vi "Autonomous Independent.vi"() -> ()   [LabVIEW 2014]
doc: "This VI is called when autonomous begins, and will automatically be terminated when autonomous ends. You can carry out timed or sensor driven robot movement independently without needing to return to the caller."
uses:
  <vilib>/Rock Robotics/WPI/RobotDrive/WPI_RobotDriveGetSetRefNum.vi
  <vilib>/Utility/file.llb/Read From Spreadsheet File (DBL).vi
  <vilib>/Rock Robotics/WPI/RobotDrive/WPI_RobotDriveMecanumDrive_Cartesian.vi
  Robot Global Data.vi
panel:
  out "?":dbl[][](array[numeric])
  out "Distance 3":dbl
  out "Distance 2":dbl
  out "Gyro Angle":dbl
  out "Gyro Angle 2":dbl
  out "Distance":bool
  out "Stop":bool
  out "Rotate":bool
  out "Shoot":bool
  out "Pick-up":bool
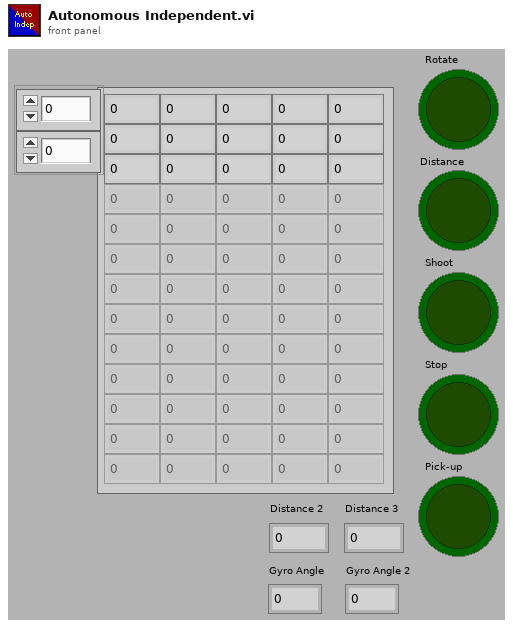
[diagram p1: front panel]
types:
  T1 = typedef "WPI_EncoderDevRef.ctl" = cluster{"DevStatus":errorcluster, "EncoderIndex":T2, "CounterIndex":T3, "DistancePerCount":dbl, "Decoding Type":T4}
  T2 = typedef "FPGA_EncoderIdx.ctl" = enum8{"Enc 0", "Enc 1", "Enc 2", "Enc 3", "Enc 4", "Enc 5", "Enc 6", "Enc 7", "Invalid"}
  T3 = typedef "FPGA_CounterCtrSystemIndex.ctl" = enum8{"Ctr 0", "Ctr 1", "Ctr 2", "Ctr 3", "Ctr 4", "Ctr 5", "Ctr 6", "Ctr 7", "Invalid"}
  T4 = typedef "WPI_EncoderType.ctl" = enum16{"1x", "2x", "4x"}
  T5 = typedef "WPI_RobotDriveDevRef.ctl" = cluster{"DevStatus":errorcluster, "Motors[]":T6[], "Square Inputs":bool, "Max Output":dbl}
  T6 = typedef "WPI_MotorControlDeviceRef.ctl" = cluster{"DeviceStatus":errorcluster, "Type":T7, "PWM":cluster{"Controller":T8, "PWM Channel":T9, "DeadBand":T10}, "CAN":cluster{"Device Number":u8, "Control Mode":T11, "Semaphore":T12, "Max Vout":dbl, "TalonSRX Control Mode":T13}, "Invert":bool, "TransformRef":T14, "InvTransformRef":T14}
  T7 = typedef "WPI_MotorControlType.ctl" = enum16{"PWM", "CAN", "CANTalonSRX"}
  T8 = typedef "FPGA_TypedefDigitalModule.ctl" = enum16{"Controller 1"}
  T9 = typedef "FPGA_DIOPWMChannel.ctl" = enum8{"PWM 0", "PWM 1", "PWM 2", "PWM 3", "PWM 4", "PWM 5", "PWM 6", "PWM 7", "PWM 8", "PWM 9", "PWM MXP 0", "PWM MXP 1", "PWM MXP 2", "PWM MXP 3", "PWM MXP 4", "PWM MXP 5", "PWM MXP 6", "PWM MXP 7", "PWM MXP 8", "PWM MXP 9", "Invalid"}
  T10 = typedef "WPI_PWMDeadband.ctl" = cluster{"Name":string, "maxPositivePwm":i32, "minPositivePwm":i32, "centerPwm":i32, "maxNegativePwm":i32, "minNegativePwm":i32, "angularRange":u16}
  T11 = typedef "WPI_CANJaguar_ControlMode.ctl" = enum8{"Percent VBus", "Current", "Speed", "Position", "Voltage"}
  T12 = typedef "Semaphore RefNum" = refnum<k1>
  T13 = typedef "WPI_CANTalonSRX_APIControlMode.ctl" = enum8{"Percent VBus", "Speed", "Position", "Slave", "Unchanged / Invalid"}
  T14 = typedef "WPI_PWMTransform_ConPane.ctl" = refnum<vi>
  T15 = typedef "WPI_GyroDevRef.ctl" = cluster{"DevStatus":errorcluster, "Analog Module":T16, "Analog Channel":T17, "Offset":dbl, "Gain (VoltsPerDegree/Second)":dbl}
  T16 = typedef "FPGA_TypedefAnalogModule.ctl" = enum16{"Controller 1"}
  T17 = typedef "FPGA_AIChannel.ctl" = enum8{"AI 0", "AI 1", "AI 2", "AI 3", "AI MXP 0", "AI MXP 1", "AI MXP 2", "AI MXP 3", "Invalid"}
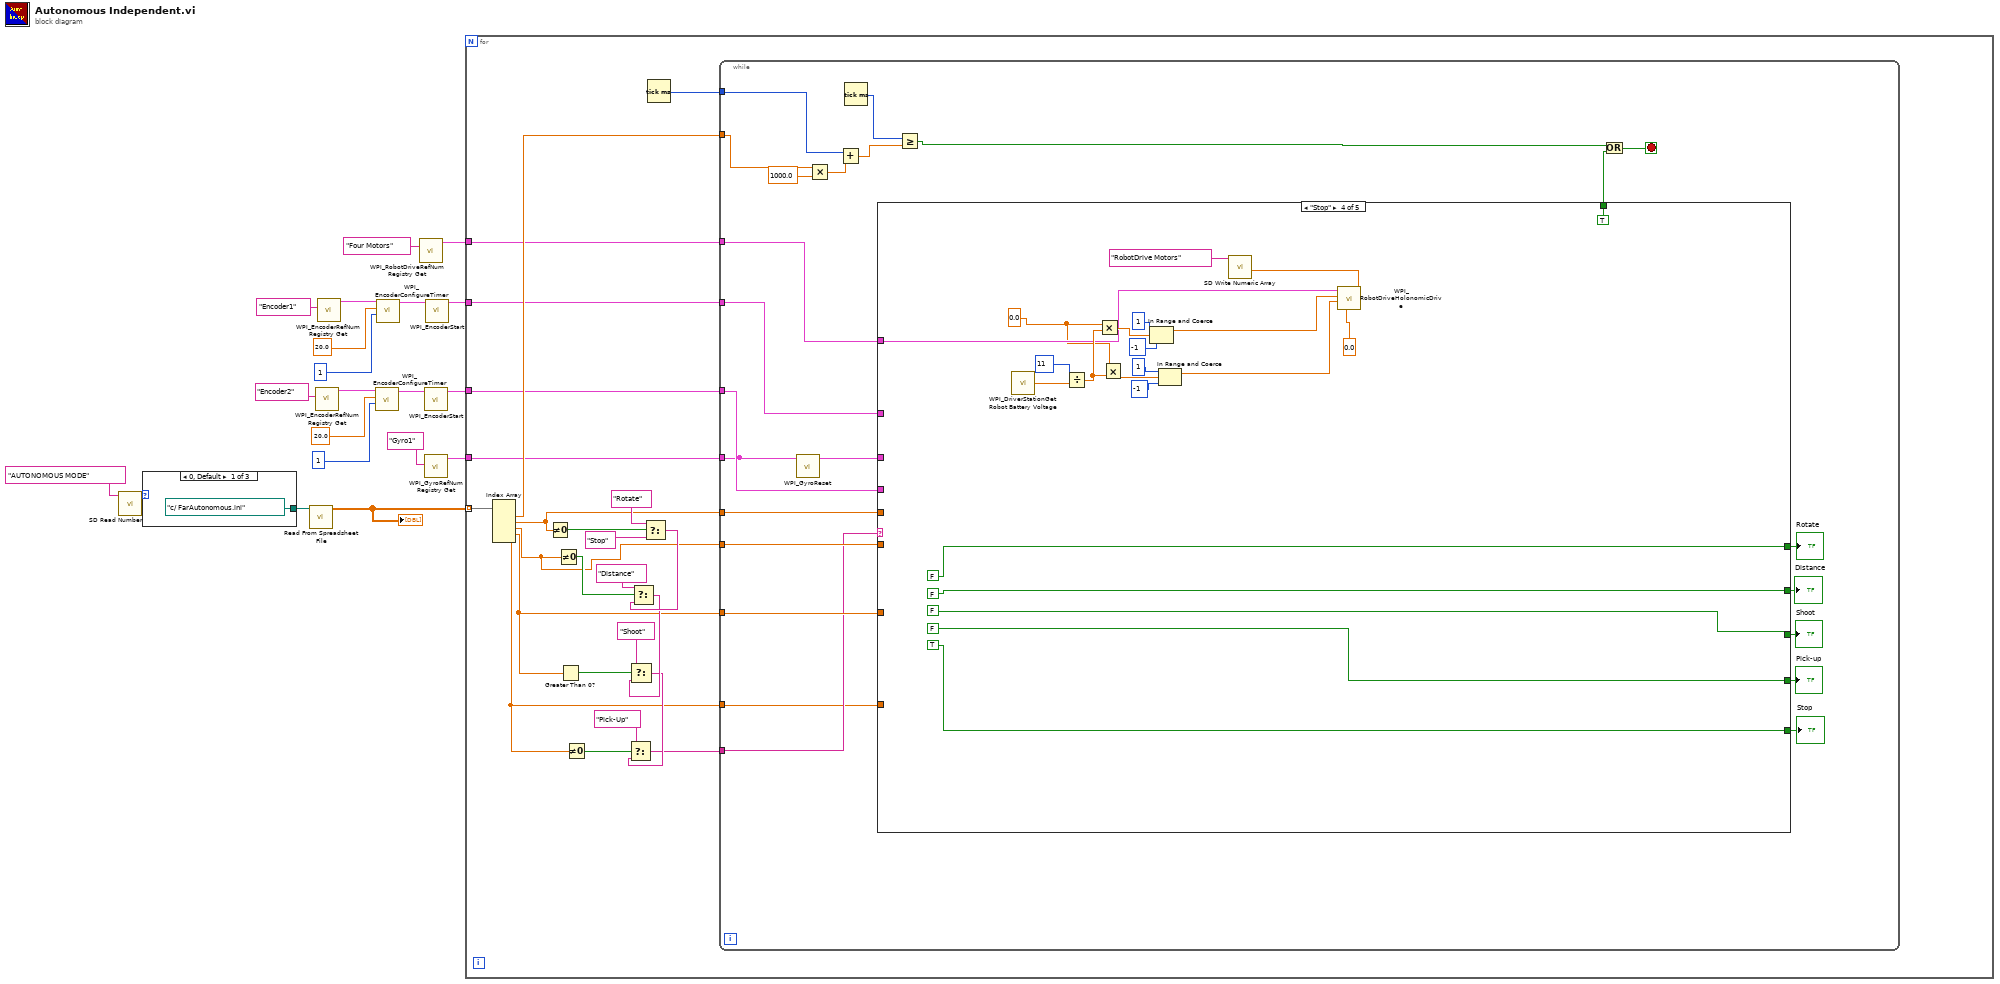
[diagram p0: block diagram]
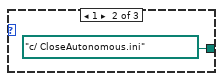
[diagram p2: hidden frame]
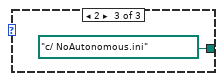
[diagram p3: hidden frame]
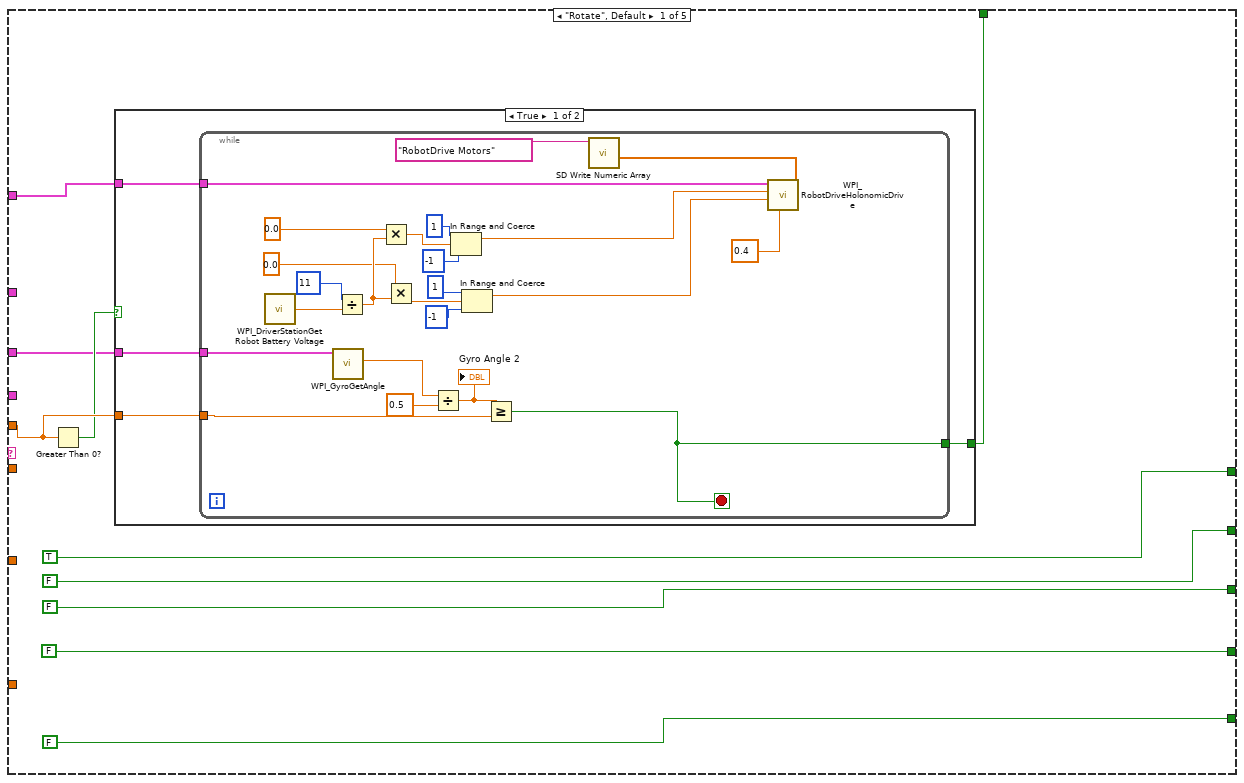
[diagram p4: hidden frame]
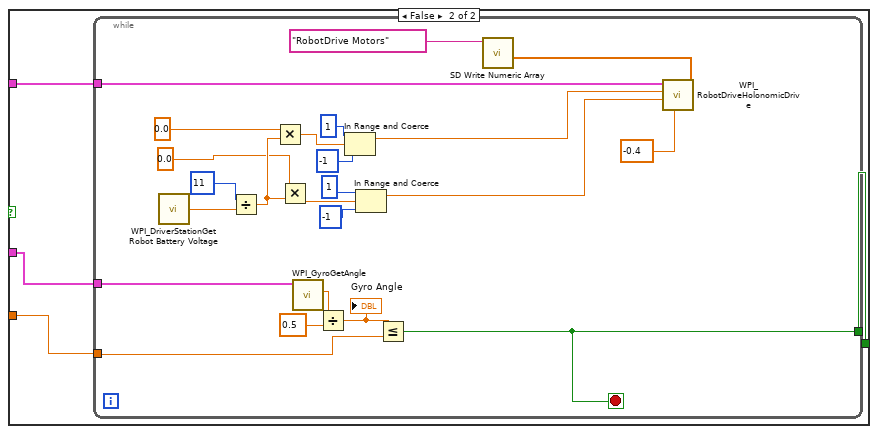
[diagram p5: hidden frame]
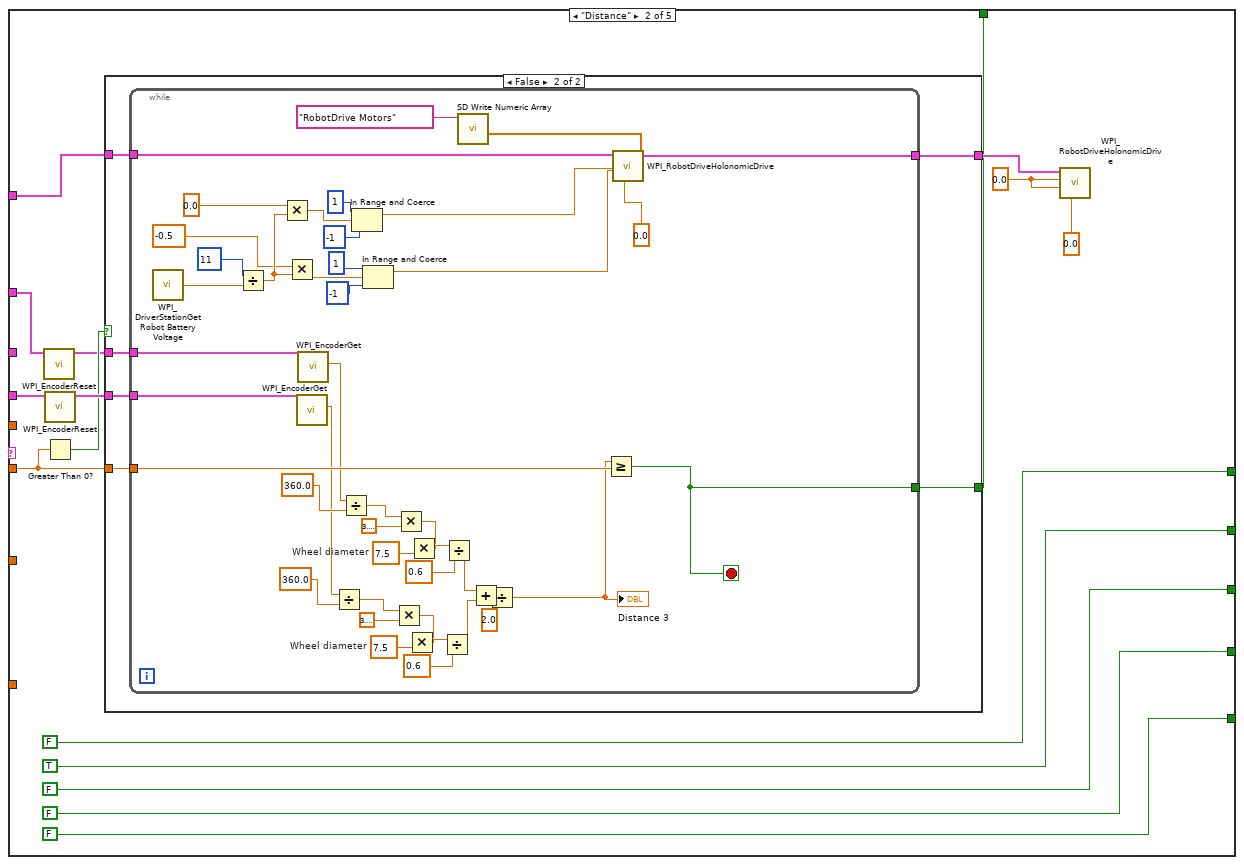
[diagram p6: hidden frame]
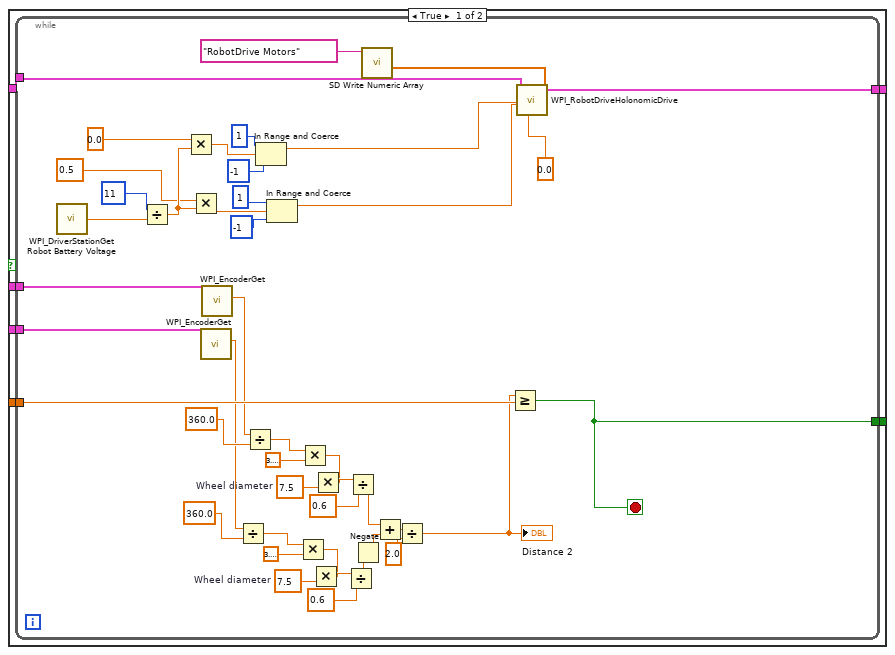
[diagram p7: hidden frame]
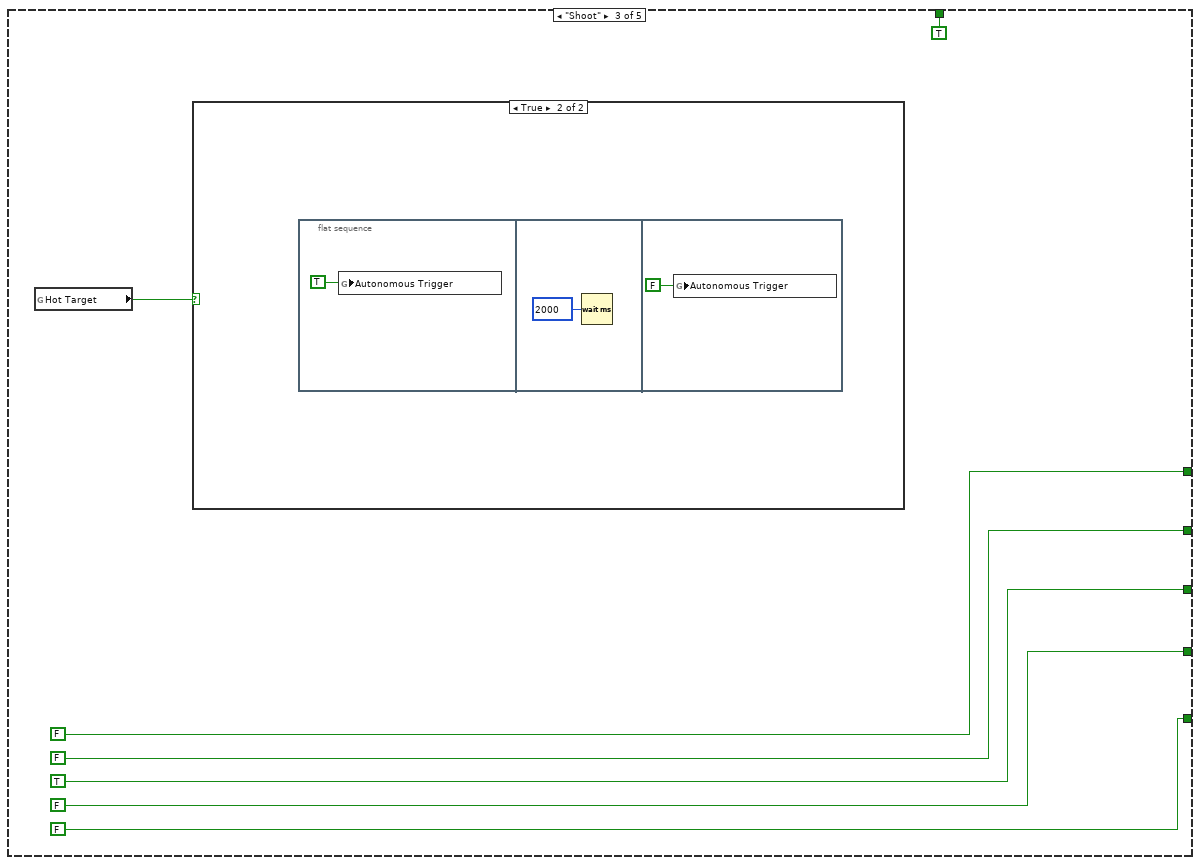
[diagram p8: hidden frame]
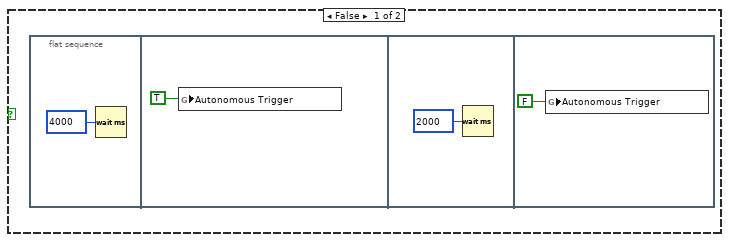
[diagram p9: hidden frame]
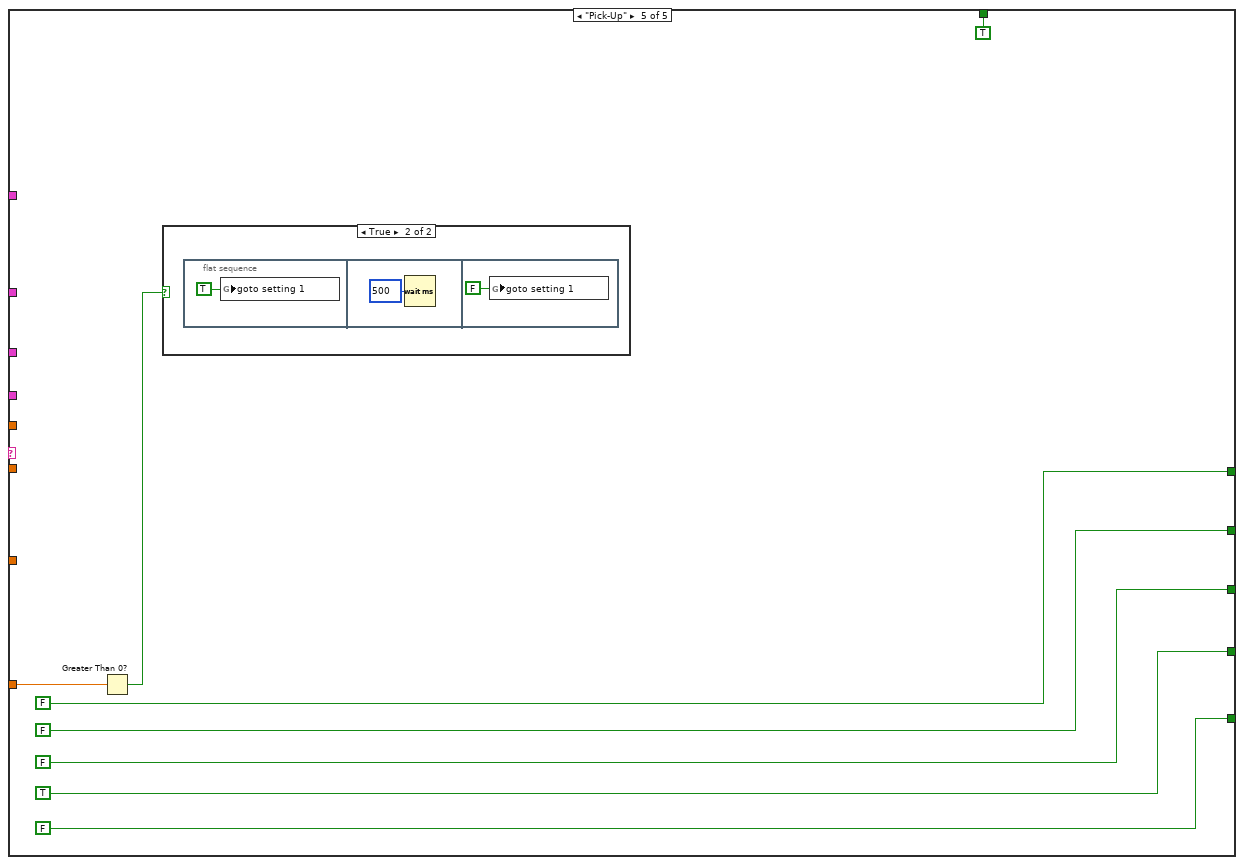
[diagram p10: hidden frame]
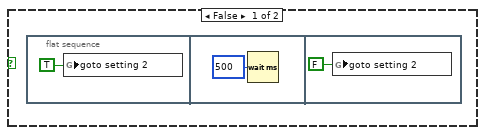
[diagram p11: hidden frame]
diagram:
  n1 = call <vilib>:"SD Read Number.vi"("Name"="AUTONOMOUS MODE") -> ("Numeric"=w2:dbl)  [unwired: 8 in, 2 out]
  n2 = case shown="0, Default" w2 {
    tunnel: [path "c:/ FarAutonomous.ini" ("file path (dialog if empty)") path "c:/ CloseAutonomous.ini" ("file path (dialog if empty)") path "c:/ NoAutonomous.ini" ("file path (dialog if empty)")] -> w4
    frame 0, Default {
    }
    frame 1 {
    }
    frame 2 {
    }
  }
  n3 = call-poly <vilib>:"Read From Spreadsheet File.vi"("file path (dialog if empty)"=w4) -> ("all rows"=w1:dbl[][])  [unwired: 6 in, 4 out]
  "?" <- w1
  n4 = call <vilib>:"WPI_EncoderRefNum Registry Get.vi"("refnum name"="Encoder2") -> ("EncoderDevRef"=w17:T1)  [unwired: 9 in, 1 out]
  n5 = call <vilib>:"WPI_EncoderRefNum Registry Get.vi"("refnum name"="Encoder1") -> ("EncoderDevRef"=w9:T1)  [unwired: 9 in, 1 out]
  n6 = call <vilib>:"WPI_EncoderConfigureTimer.vi"("Number Samples to Average"=u8 1 ("Number Samples to Average 2"), "Minimum Rate"=20.0 ("Minimum Rate 2"), "EncoderDevRef"=w17) -> ("EncoderDevRef"=w14:T1)  [unwired: 1 in, 7 out]
  n7 = call <vilib>:"WPI_EncoderConfigureTimer.vi"("Number Samples to Average"=u8 1 ("Number Samples to Average 2"), "Minimum Rate"=20.0 ("Minimum Rate 2"), "EncoderDevRef"=w9) -> ("EncoderDevRef"=w6:T1)  [unwired: 1 in, 7 out]
  n8 = call <vilib>:"WPI_RobotDriveRefNum Registry Get.vi"("refnum name"="Four Motors") -> ("RobotDriveDevRef"=w19:T5)  [unwired: 1 in, 9 out]
  n9 = call <vilib>:"WPI_EncoderStart.vi"("EncoderDevRef"=w14) -> ("EncoderDevRef"=w13:T1)  [unwired: 1 in, 9 out]
  n10 = call <vilib>:"WPI_GyroRefNum Registry Get.vi"("refnum name"="Gyro1") -> ("GyroDevRef"=w11:T15)  [unwired: 9 in, 1 out]
  n11 = call <vilib>:"WPI_EncoderStart.vi"("EncoderDevRef"=w6) -> ("EncoderDevRef"=w5:T1)  [unwired: 1 in, 9 out]
  n12 = for {
    tunnel: w1 -> [w47] mode=indexing
    tunnel: w19 -> [w36]
    tunnel: w13 -> [w35]
    tunnel: w11 -> [w33]
    tunnel: w5 -> [w29]
    n13 = Index Array(array=w47) -> (element #1=w38:dbl, element #2=w32:dbl, element #3=w34:dbl, element #4=w30:dbl, element #5=w24:dbl)  [unwired: 5 in]
    n14 = Not Equal To 0?(x=w32) -> (x != 0?=w31:bool)
    n15 = Not Equal To 0?(x=w34) -> (x != 0?=w43:bool)
    n16 = Greater Than 0?(x=w30) -> (x > 0?=w41:bool)
    n17 = Not Equal To 0?(x=w24) -> (x != 0?=w25:bool)
    n18 = Select(t="Rotate", s=w31, f="Stop") -> (s? t:f=w40:string)
    n19 = Select(t="Distance", s=w43, f=w40) -> (s? t:f=w39:string)
    n20 = Select(t="Shoot", s=w41, f=w39) -> (s? t:f=w28:string)
    n21 = Select(t="Pick-Up", s=w25, f=w28) -> (s? t:f=w26:string)
    n22 = Tick Count (ms)() -> (millisecond timer value=w37:u32)
    n23 = while {
      tunnel: w38 -> [w69]
      tunnel: w37 -> [w67]
      tunnel: w36 -> [w65]
      tunnel: w35 -> [w64]
      tunnel: w34 -> [w63]
      tunnel: [w62] -> _
      tunnel: w33 -> [w62]
      tunnel: w32 -> [w61]
      tunnel: w26 -> [w56]
      tunnel: w30 -> [w57]
      tunnel: w29 -> [w50]
      tunnel: w24 -> [w48]
      stop <- w59 stop-if-true
      n24 = call <vilib>:"WPI_GyroReset.vi"("GyroDevRef"=w62) -> ("GyroDevRef"=w51:T15)  [unwired: 9 in, 1 out]
      n25 = Multiply(x=w69, y=1000.0) -> (x*y=w68:dbl)
      n26 = Add(x=w67, y=w68) -> (x+y=w66:dbl)
      n27 = Tick Count (ms)() -> (millisecond timer value=w70:u32)
      n28 = case shown="\"Stop\"" w56 {
        tunnel: w65 -> [w81 w151 _ w273 _]
        tunnel: w64 -> [_ w148 _ _ _]
        tunnel: w63 -> [_ w145 _ _ _]
        tunnel: w51 -> [w73 _ _ _ _]
        tunnel: w61 -> [w79 _ _ _ _]
        tunnel: [w80 w146 TRUE TRUE TRUE] -> w58
        tunnel: w57 -> [_ _ _ _ _]
        tunnel: [FALSE FALSE FALSE TRUE FALSE] -> w55
        tunnel: [FALSE FALSE TRUE FALSE FALSE] -> w54
        tunnel: [FALSE TRUE FALSE FALSE FALSE] -> w53
        tunnel: [TRUE FALSE FALSE FALSE FALSE] -> w52
        tunnel: w50 -> [_ w139 _ _ _]
        tunnel: [FALSE FALSE FALSE FALSE TRUE] -> w49
        tunnel: w48 -> [_ _ _ _ w288]
        frame "Rotate", Default {
          n29 = Greater Than 0?(x=w79) -> (x > 0?=w74:bool)
          n30 = case shown="True" w74 {
            tunnel: w81 -> [w85 w112]
            tunnel: [w84 w110] -> w80
            tunnel: w79 -> [w83 w111]
            tunnel: w73 -> [w82 w109]
            frame True {
              n31 = while {
                tunnel: w85 -> [w108]
                tunnel: [w91] -> w84
                tunnel: w83 -> [w90]
                tunnel: w82 -> [w89]
                stop <- w91 stop-if-true
                n32 = call <vilib>:"WPI_DriverStationGet Robot Battery Voltage.vi"() -> ("robot battery voltage"=w105:dbl)  [unwired: 14 in, 1 out]
                n33 = call <vilib>:"WPI_GyroGetAngle.vi"("GyroDevRef"=w89) -> ("Angle"=w92:dbl)  [unwired: 7 in, 3 out]
                n34 = Divide(x=11, y=w105) -> (x/y=w103:dbl)
                n35 = Multiply(x=0.0, y=w103) -> (x*y=w100:dbl)
                n36 = Multiply(x=0.0, y=w103) -> (x*y=w99:dbl)
                n37 = Divide(x=w92, y=0.5) -> (x/y=w87:dbl)
                "Gyro Angle 2" <- w87
                n38 = In Range and Coerce(upper limit=1, x=w100, lower limit=-1) -> (coerced(x)=w96:dbl)  [unwired: 1 out]
                n39 = In Range and Coerce(upper limit=1, x=w99, lower limit=-1) -> (coerced(x)=w95:dbl)  [unwired: 1 out]
                n40 = Greater Or Equal?(x=w87, y=w90) -> (x >= y?=w91:bool)
                n41 = call-poly <vilib>:"WPI_RobotDriveHolonomicDrive.vi"("Rotation"=0.4, "Y"=w95, "X"=w96, "RobotDriveDevRef"=w108) -> ("Motor Values"=w106:dbl[])  [unwired: 5 in, 2 out]
                n42 = call <vilib>:"SD Write Numeric Array.vi"("Numeric Array"=w106, "Name"="RobotDrive Motors") -> ()  [unwired: 8 in, 2 out]
              }
            }
            frame False {
              n43 = while {
                tunnel: w112 -> [w135]
                tunnel: w111 -> [w117]
                tunnel: [w118] -> w110
                tunnel: w109 -> [w116]
                stop <- w118 stop-if-true
                n44 = call <vilib>:"WPI_DriverStationGet Robot Battery Voltage.vi"() -> ("robot battery voltage"=w132:dbl)  [unwired: 14 in, 1 out]
                n45 = Divide(x=11, y=w132) -> (x/y=w130:dbl)
                n46 = Multiply(x=0.0, y=w130) -> (x*y=w127:dbl)
                n47 = Multiply(x=0.0, y=w130) -> (x*y=w126:dbl)
                n48 = call <vilib>:"WPI_GyroGetAngle.vi"("GyroDevRef"=w116) -> ("Angle"=w119:dbl)  [unwired: 7 in, 3 out]
                n49 = Divide(x=w119, y=0.5) -> (x/y=w114:dbl)
                "Gyro Angle" <- w114
                n50 = In Range and Coerce(upper limit=1, x=w127, lower limit=-1) -> (coerced(x)=w123:dbl)  [unwired: 1 out]
                n51 = In Range and Coerce(upper limit=1, x=w126, lower limit=-1) -> (coerced(x)=w122:dbl)  [unwired: 1 out]
                n52 = Less Or Equal?(x=w114, y=w117) -> (x <= y?=w118:bool)
                n53 = call-poly <vilib>:"WPI_RobotDriveHolonomicDrive.vi"("Rotation"=-0.4, "Y"=w122, "X"=w123, "RobotDriveDevRef"=w135) -> ("Motor Values"=w133:dbl[])  [unwired: 5 in, 2 out]
                n54 = call <vilib>:"SD Write Numeric Array.vi"("Numeric Array"=w133, "Name"="RobotDrive Motors") -> ()  [unwired: 8 in, 2 out]
              }
            }
          }
        }
        frame "Distance" {
          w149 = 0.0
          n55 = call <vilib>:"WPI_EncoderReset.vi"("EncoderDevRef"=w139) -> ("EncoderDevRef"=w138:T1)  [unwired: 9 in, 1 out]
          n56 = call <vilib>:"WPI_EncoderReset.vi"("EncoderDevRef"=w148) -> ("EncoderDevRef"=w147:T1)  [unwired: 9 in, 1 out]
          n57 = Greater Than 0?(x=w145) -> (x > 0?=w144:bool)
          n58 = case shown="False" w144 {
            tunnel: w151 -> [w157 w207]
            tunnel: w145 -> [w156 w206]
            tunnel: [w155 w205] -> w150
            tunnel: w147 -> [w154 w204]
            tunnel: [w153 w203] -> w146
            tunnel: w138 -> [w152 w202]
            frame True {
              n59 = while {
                tunnel: w157 -> [w201]
                tunnel: w156 -> [w178]
                tunnel: [w200] -> w155
                tunnel: w154 -> [w199]
                tunnel: [w179] -> w153
                tunnel: w152 -> [w173]
                stop <- w179 stop-if-true
                w169 = 7.5  # Wheel diameter
                w180 = 7.5  # Wheel diameter
                n60 = call <vilib>:"WPI_DriverStationGet Robot Battery Voltage.vi"() -> ("robot battery voltage"=w196:dbl)  [unwired: 14 in, 1 out]
                n61 = Divide(x=11, y=w196) -> (x/y=w194:dbl)
                n62 = Multiply(x=0.0, y=w194) -> (x*y=w191:dbl)
                n63 = Multiply(x=0.5, y=w194) -> (x*y=w190:dbl)
                n64 = call <vilib>:"WPI_EncoderGet.vi"("EncoderDevRef"=w199) -> ("Distance"=w164:dbl)  [unwired: 5 in, 5 out]
                n65 = call <vilib>:"WPI_EncoderGet.vi"("EncoderDevRef"=w173) -> ("Distance"=w172:dbl)  [unwired: 5 in, 5 out]
                n66 = Divide(x=w164, y=360.0) -> (x/y=w165:dbl)
                n67 = Divide(x=w172, y=360.0) -> (x/y=w184:dbl)
                n68 = In Range and Coerce(upper limit=1, x=w191, lower limit=-1) -> (coerced(x)=w187:dbl)  [unwired: 1 out]
                n69 = In Range and Coerce(upper limit=1, x=w190, lower limit=-1) -> (coerced(x)=w186:dbl)  [unwired: 1 out]
                n70 = Multiply(x=w165, y=3.141592653589793) -> (x*y=w166:dbl)
                n71 = Multiply(x=w184, y=3.141592653589793) -> (x*y=w183:dbl)
                n72 = Multiply(x=w166, y=w169) -> (x*y=w170:dbl)
                n73 = Multiply(x=w183, y=w180) -> (x*y=w177:dbl)
                n74 = Divide(x=w170, y=0.6) -> (x/y=w162:dbl)
                n75 = Divide(x=w177, y=0.6) -> (x/y=w163:dbl)
                n76 = Negate(x=w162) -> (-x=w158:dbl)
                n77 = Add(x=w163, y=w158) -> (x+y=w161:dbl)
                n78 = Divide(x=w161, y=2.0) -> (x/y=w159:dbl)
                "Distance 2" <- w159
                n79 = Greater Or Equal?(x=w159, y=w178) -> (x >= y?=w179:bool)
                n80 = call-poly <vilib>:"WPI_RobotDriveHolonomicDrive.vi"("Rotation"=0.0, "Y"=w186, "X"=w187, "RobotDriveDevRef"=w201) -> ("Motor Values"=w197:dbl[], "RobotDriveDevRef"=w200:T5)  [unwired: 5 in, 1 out]
                n81 = call <vilib>:"SD Write Numeric Array.vi"("Numeric Array"=w197, "Name"="RobotDrive Motors") -> ()  [unwired: 8 in, 2 out]
              }
            }
            frame False {
              n82 = while {
                tunnel: w207 -> [w250]
                tunnel: w206 -> [w227]
                tunnel: [w249] -> w205
                tunnel: w204 -> [w248]
                tunnel: [w228] -> w203
                tunnel: w202 -> [w222]
                stop <- w228 stop-if-true
                w218 = 7.5  # Wheel diameter
                w229 = 7.5  # Wheel diameter
                n83 = call <vilib>:"WPI_DriverStationGet Robot Battery Voltage.vi"() -> ("robot battery voltage"=w245:dbl)  [unwired: 14 in, 1 out]
                n84 = Divide(x=11, y=w245) -> (x/y=w243:dbl)
                n85 = Multiply(x=0.0, y=w243) -> (x*y=w240:dbl)
                n86 = Multiply(x=-0.5, y=w243) -> (x*y=w239:dbl)
                n87 = call <vilib>:"WPI_EncoderGet.vi"("EncoderDevRef"=w248) -> ("Distance"=w213:dbl)  [unwired: 5 in, 5 out]
                n88 = call <vilib>:"WPI_EncoderGet.vi"("EncoderDevRef"=w222) -> ("Distance"=w221:dbl)  [unwired: 5 in, 5 out]
                n89 = Divide(x=w213, y=360.0) -> (x/y=w214:dbl)
                n90 = Divide(x=w221, y=360.0) -> (x/y=w233:dbl)
                n91 = In Range and Coerce(upper limit=1, x=w240, lower limit=-1) -> (coerced(x)=w236:dbl)  [unwired: 1 out]
                n92 = In Range and Coerce(upper limit=1, x=w239, lower limit=-1) -> (coerced(x)=w235:dbl)  [unwired: 1 out]
                n93 = Multiply(x=w214, y=3.141592653589793) -> (x*y=w215:dbl)
                n94 = Multiply(x=w233, y=3.141592653589793) -> (x*y=w232:dbl)
                n95 = Multiply(x=w215, y=w218) -> (x*y=w219:dbl)
                n96 = Multiply(x=w232, y=w229) -> (x*y=w226:dbl)
                n97 = Divide(x=w219, y=0.6) -> (x/y=w211:dbl)
                n98 = Divide(x=w226, y=0.6) -> (x/y=w212:dbl)
                n99 = Add(x=w212, y=w211) -> (x+y=w210:dbl)
                n100 = Divide(x=w210, y=2.0) -> (x/y=w208:dbl)
                "Distance 3" <- w208
                n101 = Greater Or Equal?(x=w208, y=w227) -> (x >= y?=w228:bool)
                n102 = call-poly <vilib>:"WPI_RobotDriveHolonomicDrive.vi"("Rotation"=0.0, "Y"=w235, "X"=w236, "RobotDriveDevRef"=w250) -> ("Motor Values"=w246:dbl[], "RobotDriveDevRef"=w249:T5)  [unwired: 5 in, 1 out]
                n103 = call <vilib>:"SD Write Numeric Array.vi"("Numeric Array"=w246, "Name"="RobotDrive Motors") -> ()  [unwired: 8 in, 2 out]
              }
            }
          }
          n104 = call-poly <vilib>:"WPI_RobotDriveHolonomicDrive.vi"("Rotation"=0.0, "Y"=w149, "X"=w149, "RobotDriveDevRef"=w150) -> ()  [unwired: 5 in, 3 out]
        }
        frame "Shoot" {
          n105 = global read "Robot Global Data.vi" "Hot Target"() -> (w253:bool)
          n106 = case shown="True" w253 {
            frame False {
              n107 = flat-sequence {
                frame #0 {
                  n108 = Wait (ms)(milliseconds to wait=u32 4000) -> ()  [unwired: 1 out]
                }
                frame #1 {
                  n109 = global write "Robot Global Data.vi" "Autonomous Trigger"(TRUE) -> ()
                }
                frame #2 {
                  n110 = Wait (ms)(milliseconds to wait=u32 2000) -> ()  [unwired: 1 out]
                }
                frame #3 {
                  n111 = global write "Robot Global Data.vi" "Autonomous Trigger"(FALSE) -> ()
                }
              }
            }
            frame True {
              n112 = flat-sequence {
                frame #0 {
                  n113 = global write "Robot Global Data.vi" "Autonomous Trigger"(TRUE) -> ()
                }
                frame #1 {
                  n114 = Wait (ms)(milliseconds to wait=u32 2000) -> ()  [unwired: 1 out]
                }
                frame #2 {
                  n115 = global write "Robot Global Data.vi" "Autonomous Trigger"(FALSE) -> ()
                }
              }
            }
          }
        }
        frame "Stop" {
          w272 = 0.0 ("x")
          n116 = call <vilib>:"WPI_DriverStationGet Robot Battery Voltage.vi"() -> ("robot battery voltage"=w284:dbl)  [unwired: 14 in, 1 out]
          n117 = Divide(x=11, y=w284) -> (x/y=w282:dbl)
          n118 = Multiply(x=w272, y=w282) -> (x*y=w279:dbl)
          n119 = Multiply(x=w272, y=w282) -> (x*y=w278:dbl)
          n120 = In Range and Coerce(upper limit=1, x=w279, lower limit=-1) -> (coerced(x)=w275:dbl)  [unwired: 1 out]
          n121 = In Range and Coerce(upper limit=1, x=w278, lower limit=-1) -> (coerced(x)=w274:dbl)  [unwired: 1 out]
          n122 = call-poly <vilib>:"WPI_RobotDriveHolonomicDrive.vi"("Rotation"=0.0, "Y"=w274, "X"=w275, "RobotDriveDevRef"=w273) -> ("Motor Values"=w285:dbl[])  [unwired: 5 in, 2 out]
          n123 = call <vilib>:"SD Write Numeric Array.vi"("Numeric Array"=w285, "Name"="RobotDrive Motors") -> ()  [unwired: 8 in, 2 out]
        }
        frame "Pick-Up" {
          n124 = Greater Than 0?(x=w288) -> (x > 0?=w287:bool)
          n125 = case shown="True" w287 {
            frame False {
              n126 = flat-sequence {
                frame #0 {
                  n127 = global write "Robot Global Data.vi" "goto setting 2"(TRUE ("goto setting 1")) -> ()
                }
                frame #1 {
                  n128 = Wait (ms)(milliseconds to wait=u32 500) -> ()  [unwired: 1 out]
                }
                frame #2 {
                  n129 = global write "Robot Global Data.vi" "goto setting 2"(FALSE ("goto setting 1")) -> ()
                }
              }
            }
            frame True {
              n130 = flat-sequence {
                frame #0 {
                  n131 = global write "Robot Global Data.vi" "goto setting 1"(TRUE ("goto setting 1")) -> ()
                }
                frame #1 {
                  n132 = Wait (ms)(milliseconds to wait=u32 500) -> ()  [unwired: 1 out]
                }
                frame #2 {
                  n133 = global write "Robot Global Data.vi" "goto setting 1"(FALSE ("goto setting 1")) -> ()
                }
              }
            }
          }
        }
      }
      "Distance" <- w53
      "Stop" <- w55
      "Rotate" <- w52
      "Shoot" <- w54
      "Pick-up" <- w49
      n134 = Greater Or Equal?(x=w70, y=w66) -> (x >= y?=w60:bool)
      n135 = Or(x=w60, y=w58) -> (x .or. y?=w59:bool)
    }
  }
